vi "PythonOpenTCP.vi"(0 "directory":path, 4 "debug":bool, 5 "script name":string="localhost", 6 "launch_python":bool, 8 "timeout in":i32=-1, 11 "arguments":string="localhost") -> (1 "error out":errorcluster, 2 "connection out":refnum<k5>, 3 "standard error":string, 10 "timeout out":i32, 12 "run_tcp":bool, 14 "standard output":string)   [LabVIEW 2014]
panel:
  out "command line":string
  out "return code":i32
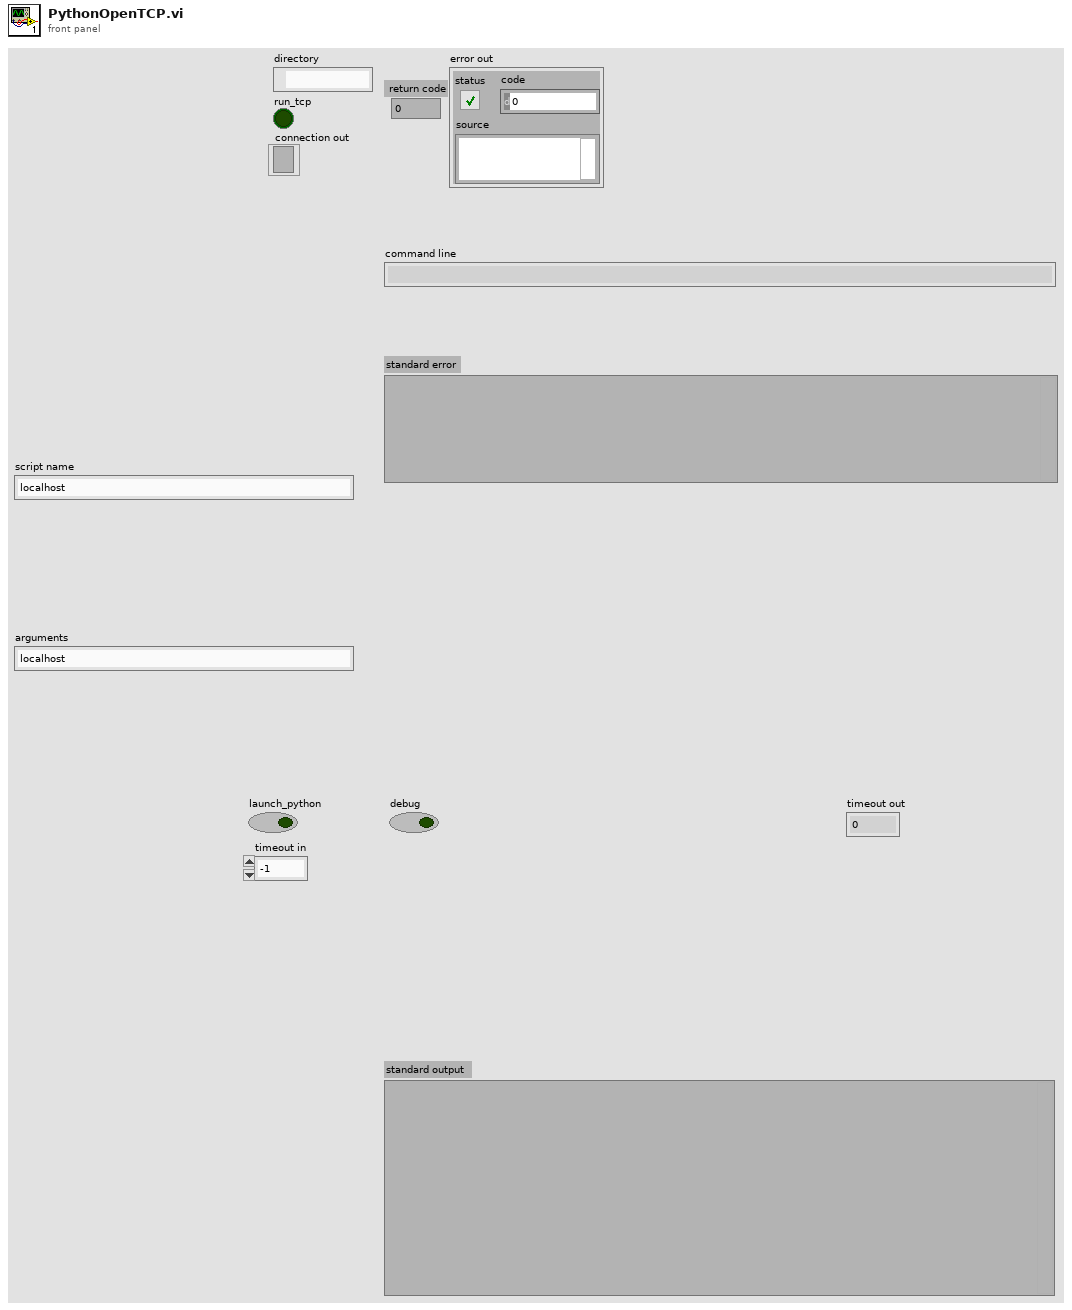
[diagram p1: front panel]
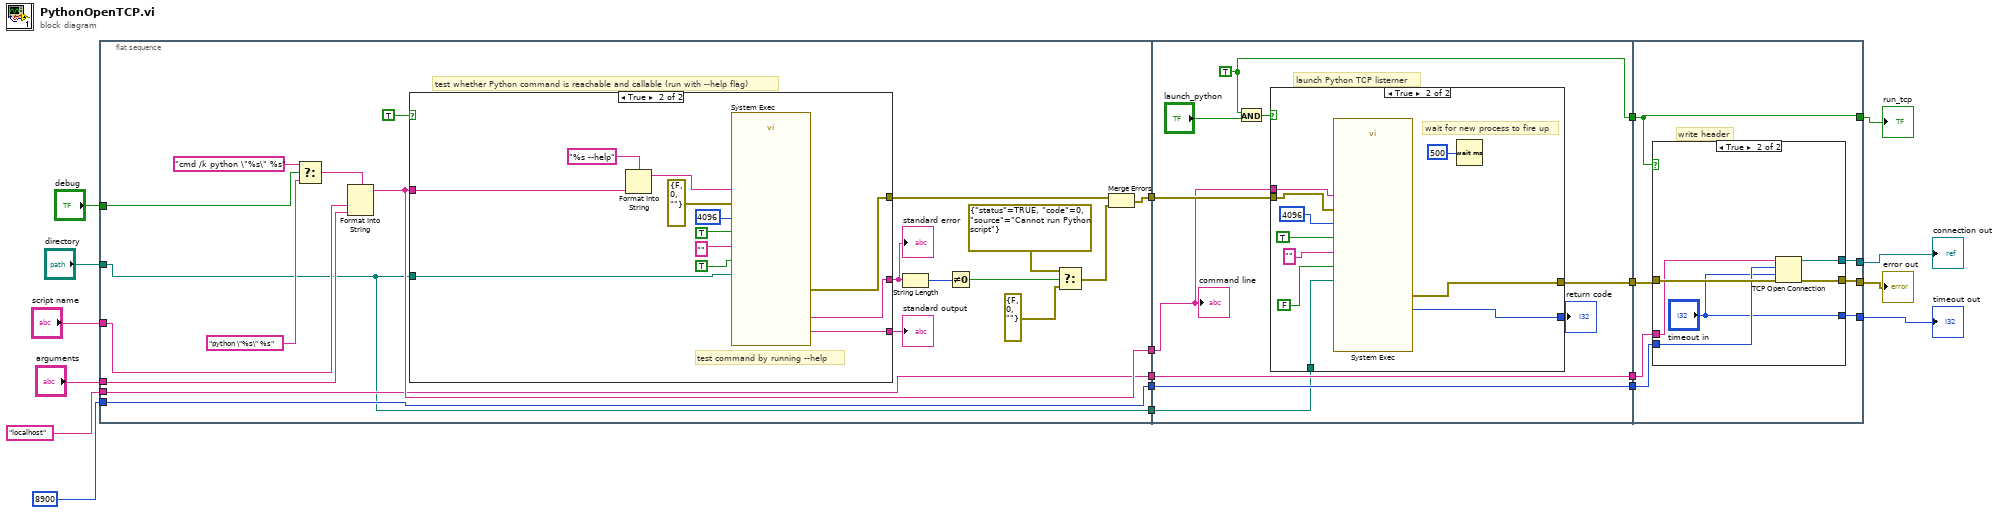
[diagram p0: block diagram]
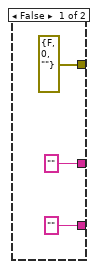
[diagram p2: hidden frame]
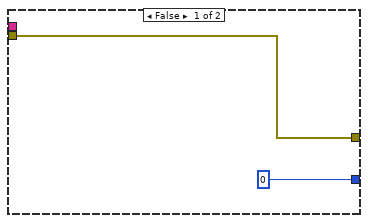
[diagram p3: hidden frame]
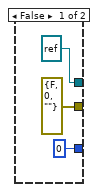
[diagram p4: hidden frame]
diagram:
  n1 = flat-sequence {
    tunnel: [w37] -> w19
    tunnel: [w31] -> w18
    tunnel: "directory" -> [w20]
    tunnel: "script name" -> [w24]
    tunnel: "arguments" -> [w23]
    tunnel: "localhost" ("hostname") -> [w22]
    tunnel: 8900 ("port") -> [w21]
    tunnel: [w21] -> w6
    tunnel: [w22] -> w4
    tunnel: "debug" -> [w34]
    tunnel: [w20] -> w1
    tunnel: [w58] -> w17
    tunnel: w19 -> [w56]
    tunnel: w18 -> [w63]
    tunnel: [w62] -> w16
    tunnel: [w61] -> w7
    tunnel: w6 -> [w61]
    tunnel: [w60] -> w5
    tunnel: w4 -> [w60]
    tunnel: w1 -> [w55]
    tunnel: [w78] -> w10
    tunnel: [w82] -> w9
    tunnel: [w81] -> w8
    tunnel: [w77] -> w2
    tunnel: w5 -> [w79]
    tunnel: w7 -> [w80]
    tunnel: w16 -> [w83]
    tunnel: w17 -> [w78]
    frame #0 {
      # "test whether Python command is reachable and callable (run with --help flag)"
      n2 = Select(t="cmd /k python \"%s\" %s" ("command line"), s=w34, f="python \"%s\" %s" ("command line")) -> (s? t:f=w25:string)
      n3 = Format Into String(format string=w25, w24, w23) -> (resulting string=w37:string)  [unwired: 2 in, 1 out]
      n4 = case shown="True" TRUE {
        tunnel: w37 -> [_ w48]
        tunnel: ["" ("standard error") w47] -> w36
        tunnel: ["" ("standard output") w46] -> w38
        tunnel: [errorcluster {"status"=FALSE, "code"=0, "source"=""} ("error out") w45] -> w30
        tunnel: w20 -> [_ w43]
        frame False {
        }
        frame True {
          # "test command by running --help"
          n5 = Format Into String(format string="%s --help" ("command line"), w48) -> (resulting string=w54:string)  [unwired: 2 in, 1 out]
          n6 = call <vilib>:"System Exec.vi"("expected output size  (4096)"=u32 4096, "run minimized? (F)"=TRUE, "wait until completion? (T)"=TRUE, "error in (no error)"=errorcluster {"status"=FALSE, "code"=0, "source"=""}, "working directory"=w43, "standard input"="", "command line"=w54) -> ("error out"=w45:errorcluster, "standard error"=w47:string, "standard output"=w46:string)  [unwired: 1 in, 1 out]
        }
      }
      "standard error" <- w36
      "standard output" <- w38
      n7 = String Length(string=w36) -> (length=w35:i32)
      n8 = Not Equal To 0?(x=w35) -> (x != 0?=w29:bool)
      n9 = Select(t=errorcluster {"status"=TRUE, "code"=0, "source"="Cannot run Python script"} ("error out"), s=w29, f=errorcluster {"status"=FALSE, "code"=0, "source"=""} ("error out")) -> (s? t:f=w26:errorcluster)
      n10 = Merge Errors(w30, w26) -> (w31:errorcluster)
    }
    frame #1 {
      w58 = TRUE
      # "launch Python TCP listerner"
      n11 = And(x=w58, y="launch_python") -> (x .and. y?=w59:bool)
      n12 = case shown="True" w59 {
        tunnel: [0 ("return code") w72] -> w64
        tunnel: w63 -> [w65 w71]
        tunnel: [w65 w70] -> w62
        tunnel: w56 -> [_ w68]
        tunnel: w55 -> [_ w67]
        frame False {
        }
        frame True {
          # "wait for new process to fire up"
          n13 = call <vilib>:"System Exec.vi"("expected output size  (4096)"=u32 4096, "run minimized? (F)"=TRUE, "wait until completion? (T)"=FALSE, "error in (no error)"=w71, "working directory"=w67, "standard input"="", "command line"=w68) -> ("error out"=w70:errorcluster, "return code"=w72:i32)  [unwired: 1 in, 2 out]
          n14 = Wait (ms)(milliseconds to wait=u32 500) -> ()  [unwired: 1 out]
        }
      }
      "return code" <- w64
      "command line" <- w56
    }
    frame #2 {
      # "write header"
      n15 = case shown="True" w78 {
        tunnel: w83 -> [_ w92]
        tunnel: [refnum<k5> refnum ("connection ID") w91] -> w82
        tunnel: [errorcluster {"status"=FALSE, "code"=0, "source"=""} ("error out") w90] -> w81
        tunnel: w80 -> [_ w89]
        tunnel: w79 -> [_ w88]
        tunnel: [0 ("timeout ms (60000)") "timeout in"] -> w77
        frame False {
        }
        frame True {
          n16 = TCP Open Connection(address=w88, remote port or service name=w89, timeout ms (60000)="timeout in", error in (no error)=w92) -> (connection ID=w91:refnum<k5>, error out=w90:errorcluster)  [unwired: 1 in]
        }
      }
    }
  }
  "run_tcp" <- w10
  "connection out" <- w9
  "error out" <- w8
  "timeout out" <- w2
